vi "Custom_Create_VI_Documentation_Component_MultiImages.vi"(6 "special chars in file path of image":string, 7 "Content Options":T1, 8 "error in (no error)":errorcluster, 9 "Image Depth":i32=24, 10 "Image Format (jpeg)":enum32{"PNG", "JPEG", "GIF"}(ring)=enum."JPEG", 11 "VI":refnum<vi>) -> (0 "error out":errorcluster, 3 "Paths to images":path[](array[path]))   [LabVIEW 2019]
uses:
  <vilib>/printing/ReportDocExtensions.llb/File_types_for_reports.ctl
  <vilib>/Utility/NIReport.llb/NI_ReportGenerationCore.lvlib
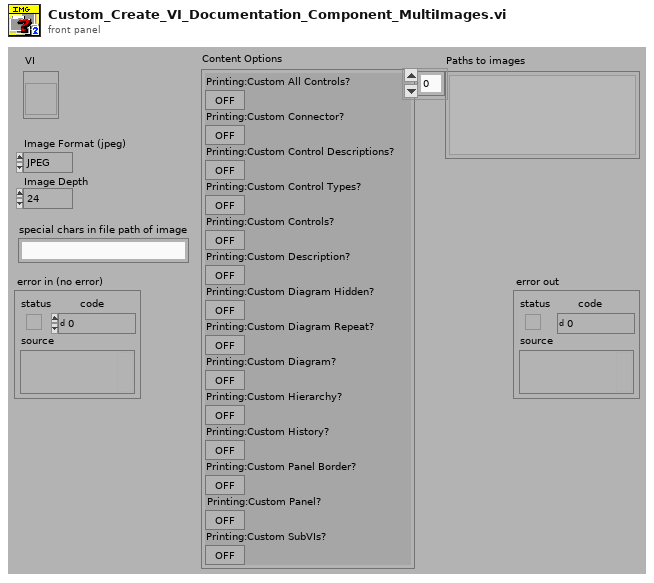
[diagram p1: front panel]
types:
  T1 = cluster{"Printing:Custom All Controls?":bool, "Printing:Custom Connector?":bool, "Printing:Custom Control Descriptions?":bool, "Printing:Custom Control Types?":bool, "Printing:Custom Controls?":bool, "Printing:Custom Description?":bool, "Printing:Custom Diagram Hidden?":bool, "Printing:Custom Diagram Repeat?":bool, "Printing:Custom Diagram?":bool, "Printing:Custom Hierarchy?":bool, "Printing:Custom History?":bool, "Printing:Custom Panel Border?":bool, "Printing:Custom Panel?":bool, "Printing:Custom SubVIs?":bool}
  T2 = typedef "NI_ReportGenerationCore.lvlib/File_types_for_reports.ctl" = enum16{".jpg", ".png", ".html", ".gif"}
  T3 = enum32{"Custom", "Standard", "Using Panel", "Using SubVI", "Complete"}
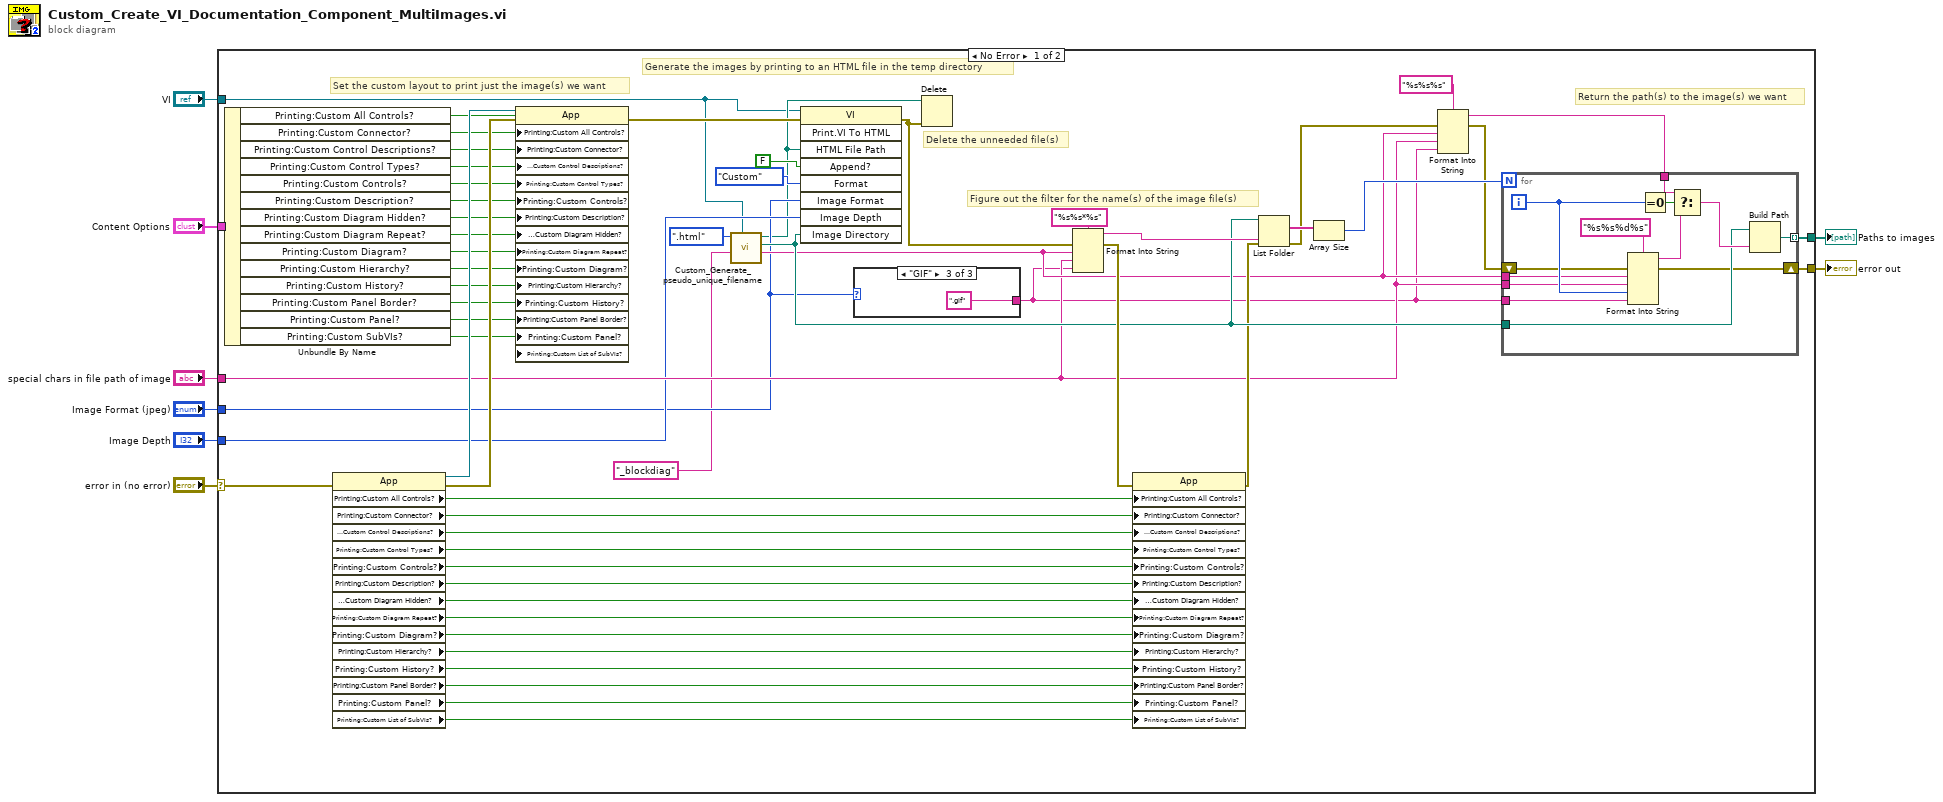
[diagram p0: block diagram]
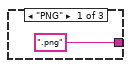
[diagram p2: hidden frame]
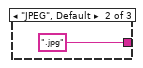
[diagram p3: hidden frame]
diagram:
  n1 = case shown="No Error" "error in (no error)" {
    selector: "error in (no error)" -> [w14 w83]
    tunnel: "VI" -> [w10 _]
    tunnel: "Content Options" -> [w43 _]
    tunnel: "special chars in file path of image" -> [w21 _]
    tunnel: [w18 _] -> w5
    tunnel: [w15 w83] -> w4
    tunnel: "Image Depth" -> [w13 _]
    tunnel: "Image Format (jpeg)" -> [w12 _]
    frame No Error {
      # "Figure out the filter for the name(s) of the image file(s)"
      # "Return the path(s) to the image(s) we want"
      # "Delete the unneeded file(s)"
      # "Generate the images by printing to an HTML file in the temp directory"
      # "Set the custom layout to print just the image(s) we want"
      n2 = Unbundle By Name(w43) -> ("Printing:Custom All Controls?"=w42:bool, "Printing:Custom Connector?"=w41:bool, "Printing:Custom Control Descriptions?"=w40:bool, "Printing:Custom Control Types?"=w39:bool, "Printing:Custom Controls?"=w38:bool, "Printing:Custom Description?"=w37:bool, "Printing:Custom Diagram Hidden?"=w36:bool, "Printing:Custom Diagram Repeat?"=w35:bool, "Printing:Custom Diagram?"=w34:bool, "Printing:Custom Hierarchy?"=w33:bool, "Printing:Custom History?"=w32:bool, "Printing:Custom Panel Border?"=w31:bool, "Printing:Custom Panel?"=w30:bool, "Printing:Custom SubVIs?"=w29:bool)
      n3 = property class="App"(error in=w14) -> (reference out=w52:refnum<vi>, error out=w51:errorcluster, "Printing:Custom All Controls?"=w53:bool, "Printing:Custom Connector?"=w54:bool, "Printing:Custom Control Descriptions?"=w55:bool, "Printing:Custom Control Types?"=w56:bool, "Printing:Custom Controls?"=w57:bool, "Printing:Custom Description?"=w58:bool, "Printing:Custom Diagram Hidden?"=w59:bool, "Printing:Custom Diagram Repeat?"=w60:bool, "Printing:Custom Diagram?"=w61:bool, "Printing:Custom Hierarchy?"=w62:bool, "Printing:Custom History?"=w63:bool, "Printing:Custom Panel Border?"=w64:bool, "Printing:Custom Panel?"=w65:bool, "Printing:Custom List of SubVIs?"=w66:bool)  [unwired: 1 in]
      n4 = property class="App"(reference=w52, error in=w51, "Printing:Custom All Controls?"=w42, "Printing:Custom Connector?"=w41, "Printing:Custom Control Descriptions?"=w40, "Printing:Custom Control Types?"=w39, "Printing:Custom Controls?"=w38, "Printing:Custom Description?"=w37, "Printing:Custom Diagram Hidden?"=w36, "Printing:Custom Diagram Repeat?"=w35, "Printing:Custom Diagram?"=w34, "Printing:Custom Hierarchy?"=w33, "Printing:Custom History?"=w32, "Printing:Custom Panel Border?"=w31, "Printing:Custom Panel?"=w30, "Printing:Custom List of SubVIs?"=w29) -> (error out=w50:errorcluster)  [unwired: 1 out]
      n5 = call "Custom_Generate_pseudo_unique_filename.vi"("VI"=w10, "Suffix"="_blockdiag", "file type(.jpg)"=File_types_for_reports.".html") -> ("root filename"=w22:string, "temp directory"=w25:path, "generated path"=w11:path)  [unwired: 6 in]
      n6 = invoke class="VI" method="Print.VI To HTML"(reference=w10, error in=w50, "HTML File Path"=w11, "Append?"=FALSE, "Format"=T3."Custom", "Image Format"=w12, "Image Depth"=w13, "Image Directory"=w25) -> (error out=w44:errorcluster)  [unwired: 1 in, 8 out]
      n7 = case shown="\"GIF\"" w12 {
        tunnel: [".png" ".jpg" ".gif"] -> w20
        frame "PNG" {
        }
        frame "JPEG", Default {
        }
        frame "GIF" {
        }
      }
      n8 = Delete(path (use dialog)=w11, error in=w44) -> ()  [unwired: 3 in, 3 out]
      n9 = Format Into String(format string="%s%s*%s" ("Format String"), error in=w44, w22, w21, w20) -> (resulting string=w28:string, error out=w45:errorcluster)  [unwired: 1 in]
      n10 = property class="App"(error in=w45, "Printing:Custom All Controls?"=w53, "Printing:Custom Connector?"=w54, "Printing:Custom Control Descriptions?"=w55, "Printing:Custom Control Types?"=w56, "Printing:Custom Controls?"=w57, "Printing:Custom Description?"=w58, "Printing:Custom Diagram Hidden?"=w59, "Printing:Custom Diagram Repeat?"=w60, "Printing:Custom Diagram?"=w61, "Printing:Custom Hierarchy?"=w62, "Printing:Custom History?"=w63, "Printing:Custom Panel Border?"=w64, "Printing:Custom Panel?"=w65, "Printing:Custom List of SubVIs?"=w66) -> (error out=w24:errorcluster)  [unwired: 1 in, 1 out]
      n11 = List Folder(path=w25, pattern=w28, error in=w24) -> (filenames=w27:string[], error out=w17:errorcluster)  [unwired: 1 in, 2 out]
      n12 = Array Size(array=w27) -> (size(s)=w26:i32)
      n13 = Format Into String(format string="%s%s%s", error in=w17, w22, w21, w20) -> (resulting string=w19:string, error out=w16:errorcluster)  [unwired: 1 in]
      n14 = for {
        N: w26 -> [_]
        tunnel: w25 -> [w70]
        tunnel: w22 -> [w73]
        tunnel: w21 -> [w74]
        tunnel: w20 -> [w75]
        tunnel: w19 -> [w72]
        tunnel: [w69] -> w18 mode=indexing
        shift-right: [w67] -> w15
        shift-left: w16 -> [w68]
        i -> [w77]
        n15 = Format Into String(format string="%s%s%d%s", error in=w68, w73, w74, w77, w75) -> (resulting string=w76:string, error out=w67:errorcluster)  [unwired: 1 in]
        n16 = Equal To 0?(x=w77) -> (x = 0?=w78:bool)
        n17 = Select(t=w72, s=w78, f=w76) -> (s? t:f=w71:string)
        n18 = Build Path(base path=w70, name or relative path=w71) -> (appended path=w69:path)
      }
    }
    frame Error {
    }
  }
  "error out" <- w4
  "Paths to images" <- w5
